vi "Configure Integration.vi"(7 "Integration Time (1 PLCs)":dbl=1.0, 8 "error in (no error)":errorcluster, 9 "Auto Integration (0: OFF)":i32(ring) items=["OFF", "ON", "ONCE"], 10 "Measurement Function (0: Voltage)":i32(ring) items=["Voltage", "Current", "Resistance", "Charge"], 11 "VISA resource name":refnum<visa-resource-name>) -> (0 "error out":errorcluster, 3 "VISA resource name out":refnum<visa-resource-name>)   [LabVIEW 2020, in "Keithley 6517.lvlib"]
doc: "Configures the integration settings for the measurement functions (Voltage, Current., Resistance and Charge).\n\nNotes:\n(1) The integration period (measurement speed) for the Model 6517B can be set using either of two commands: NPLCycle or :APERture. The NPLC method specifies the integration period as the number of power line cycles per integration, while aperture specifies the time (in seconds) per integration. The relationship between NPLC and aperture is expressed as follows:\nAperture = NPLC/f\nWhere:\nAperture is the integration rate in seconds per integration.\nNPLC is the number of power line cycles per integration.\nf is the power line frequency.\n(2) APERture commands that can be configured in <b> Configure Aperture.vi .</b>\n(3)The specified measurement should be enabled from <b>Configure Measurement Function.vi</b>.\n(4)Auto Integration is NOT available for <B>model 6514</B>."
uses:
  <instrlib>/Keithley 6517/Keithley 6517.lvlib
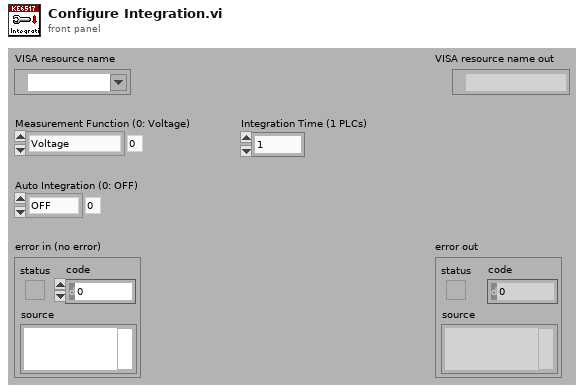
[diagram p1: front panel]
types:
  T1 = typedef "Keithley 6517.lvlib/Extended User Data.ctl" = cluster{"Instrument Model":i32}
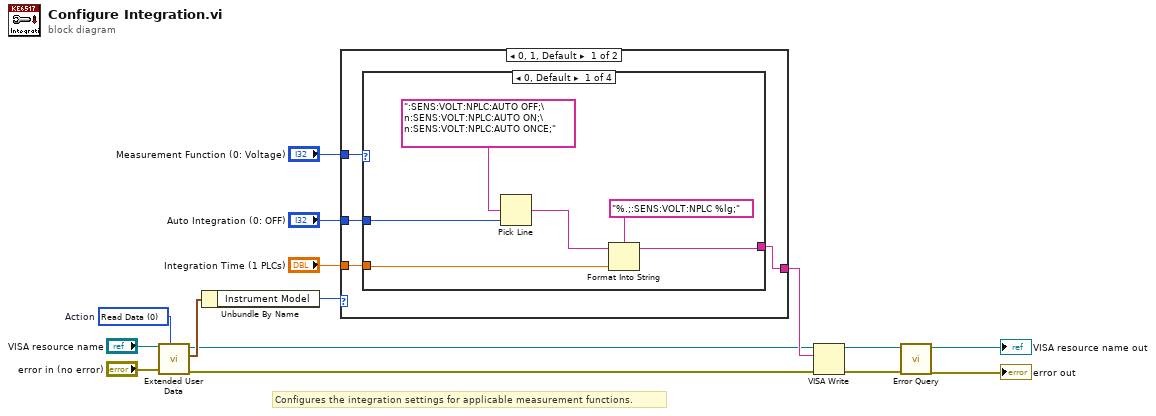
[diagram p0: block diagram]
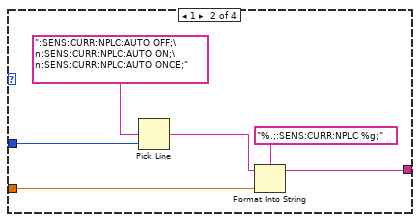
[diagram p2: hidden frame]
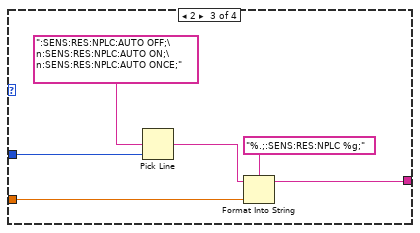
[diagram p3: hidden frame]
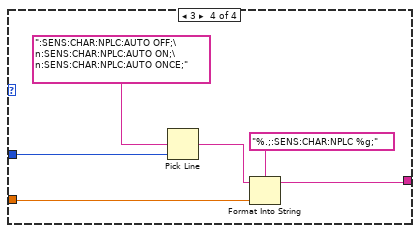
[diagram p4: hidden frame]
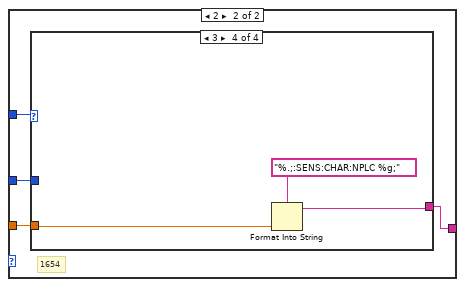
[diagram p5: hidden frame]
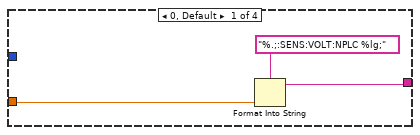
[diagram p6: hidden frame]
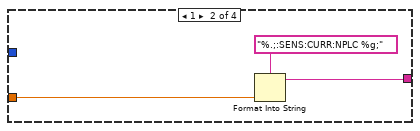
[diagram p7: hidden frame]
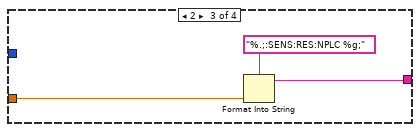
[diagram p8: hidden frame]
diagram:
  w1 = u16 0 items=["Read Data", "Write Data", "Clear Data", "Clear ALL Data"]  # Action
  # "Configures the integration settings for applicable measurement functions."
  n1 = call <instrlib>:"Extended User Data.vi"("Action (0: Read Data)"=w1, "error in (no error)"="error in (no error)", "VISA resource name"="VISA resource name") -> ("error out"=w3:errorcluster, "User Data Out"=w5:T1, "VISA resource name out"=w2:refnum<visa-resource-name>)  [unwired: 6 in]
  n2 = Unbundle By Name(w5) -> ("Instrument Model"=w4:i32)
  n3 = case shown="0, 1, Default" w4 {
    tunnel: "Auto Integration (0: OFF)" -> [w19 w47]
    tunnel: "Integration Time (1 PLCs)" -> [w18 w46]
    tunnel: [w17 w44] -> w9
    tunnel: "Measurement Function (0: Voltage)" -> [w16 w45]
    frame 0, 1, Default {
      n4 = case shown="0, Default" w16 {
        tunnel: w19 -> [w24 w30 w36 w40]
        tunnel: w18 -> [w21 w27 w33 w39]
        tunnel: [w20 w26 w32 w38] -> w17
        frame 0, Default {
          n5 = Pick Line(multi-line string=":SENS:VOLT:NPLC:AUTO OFF;\n:SENS:VOLT:NPLC:AUTO ON;\n:SENS:VOLT:NPLC:AUTO ONCE;", line index=w24) -> (output string=w22:string)  [unwired: 1 in]
          n6 = Format Into String(format string="%.;:SENS:VOLT:NPLC %lg;", initial string=w22, w21) -> (resulting string=w20:string)  [unwired: 1 in, 1 out]
        }
        frame 1 {
          n7 = Pick Line(multi-line string=":SENS:CURR:NPLC:AUTO OFF;\n:SENS:CURR:NPLC:AUTO ON;\n:SENS:CURR:NPLC:AUTO ONCE;", line index=w30) -> (output string=w28:string)  [unwired: 1 in]
          n8 = Format Into String(format string="%.;:SENS:CURR:NPLC %g;", initial string=w28, w27) -> (resulting string=w26:string)  [unwired: 1 in, 1 out]
        }
        frame 2 {
          n9 = Pick Line(multi-line string=":SENS:RES:NPLC:AUTO OFF;\n:SENS:RES:NPLC:AUTO ON;\n:SENS:RES:NPLC:AUTO ONCE;", line index=w36) -> (output string=w34:string)  [unwired: 1 in]
          n10 = Format Into String(format string="%.;:SENS:RES:NPLC %g;", initial string=w34, w33) -> (resulting string=w32:string)  [unwired: 1 in, 1 out]
        }
        frame 3 {
          n11 = Pick Line(multi-line string=":SENS:CHAR:NPLC:AUTO OFF;\n:SENS:CHAR:NPLC:AUTO ON;\n:SENS:CHAR:NPLC:AUTO ONCE;", line index=w40) -> (output string=w42:string)  [unwired: 1 in]
          n12 = Format Into String(format string="%.;:SENS:CHAR:NPLC %g;", initial string=w42, w39) -> (resulting string=w38:string)  [unwired: 1 in, 1 out]
        }
      }
    }
    frame 2 {
      # "1654"
      n13 = case shown="3" w45 {
        tunnel: w47 -> [_ _ _ _]
        tunnel: w46 -> [w49 w52 w55 w58]
        tunnel: [w48 w51 w54 w57] -> w44
        frame 0, Default {
          n14 = Format Into String(format string="%.;:SENS:VOLT:NPLC %lg;", w49) -> (resulting string=w48:string)  [unwired: 2 in, 1 out]
        }
        frame 1 {
          n15 = Format Into String(format string="%.;:SENS:CURR:NPLC %g;", w52) -> (resulting string=w51:string)  [unwired: 2 in, 1 out]
        }
        frame 2 {
          n16 = Format Into String(format string="%.;:SENS:RES:NPLC %g;", w55) -> (resulting string=w54:string)  [unwired: 2 in, 1 out]
        }
        frame 3 {
          n17 = Format Into String(format string="%.;:SENS:CHAR:NPLC %g;", w58) -> (resulting string=w57:string)  [unwired: 2 in, 1 out]
        }
      }
    }
  }
  n18 = VISA Write(VISA resource name=w2, write buffer=w9, error in (no error)=w3) -> (VISA resource name out=w15:refnum<visa-resource-name>, error out=w14:errorcluster)  [unwired: 1 out]
  n19 = call <instrlib>:"Error Query.vi"("error in (no error)"=w14, "VISA resource name"=w15) -> ("error out"=→"error out":errorcluster, "VISA resource name out"=→"VISA resource name out":refnum<visa-resource-name>)  [unwired: 6 in, 2 out]
